vi "IR_OPO_Capture_V2.vi"(0 "Commands array":string[][](array[string])=[["Group20.825", "Group20.671", "Group20.814", "Group30.121"], ["Group2-0.528", "Group2-1.243", "Group2-0.539", "Group30.121"], ["Group20.374", "Group21.573", "Group20.363", "Group30.121"], ["Group2-0.242", "Group2-1.815", "Group2-0.253", "Group30.121"], ["Group20.165", "Group21.991", "Group20.154", "Group30.121"], ["Group2-0.077", "Group2-2.145", "Group2-0.088", "Group30.121"], ["Group20.044", "Group22.233", "Group20.033", "Group30.121"], ["Group2-2.310", "WT10", "WT10", "Group30.121"], ["Group22.310", "WT10", "WT10", "Group30.121"], ["Group2-2.310", "WT10", "WT10", "Group30.121"], ["Group22.310", "WT10", "WT10", "Group30.121"], ["Group2-2.310", "WT10", "WT10", "Group30.121"], ["Group22.310", "WT10", "WT10", "Group30.121"], ["Group2-0.011", "Group2-2.277", "Group2-0.022", "Group30.121"], ["Group20.066", "Group22.189", "Group20.055", "Group30.121"], ["Group2-0.121", "Group2-2.057", "Group2-0.132", "Group30.121"], ["Group20.209", "Group21.903", "Group20.198", "Group30.121"], ["Group2-0.297", "Group2-1.705", "Group2-0.308", "Group30.121"], ["Group20.451", "Group21.419", "Group20.440", "Group30.121"], ["Group2-0.660", "Group2-0.979", "Group2-0.671", "Group30.121"]], 1 "XPS_Address":string="192.168.254.254", 2 "VISA resource name":refnum<visa-resource-name>, 3 "laser array index":i32, 4 "Process time":dbl format="%#_13g", 5 "Axis Speed":dbl=1.0 format="%#_13g", 6 "Laser on/off array":bool[][](array[boolean])=[[FALSE, TRUE, FALSE, FALSE], [FALSE, TRUE, FALSE, FALSE], [FALSE, TRUE, FALSE, FALSE], [FALSE, TRUE, FALSE, FALSE], [FALSE, TRUE, FALSE, FALSE], [FALSE, TRUE, FALSE, FALSE], [FALSE, TRUE, FALSE, FALSE], [TRUE, FALSE, FALSE, FALSE], [TRUE, FALSE, FALSE, FALSE], [TRUE, FALSE, FALSE, FALSE], [TRUE, FALSE, FALSE, FALSE], [TRUE, FALSE, FALSE, FALSE], [TRUE, FALSE, FALSE, FALSE], [FALSE, TRUE, FALSE, FALSE], [FALSE, TRUE, FALSE, FALSE], [FALSE, TRUE, FALSE, FALSE], [FALSE, TRUE, FALSE, FALSE], [FALSE, TRUE, FALSE, FALSE], [FALSE, TRUE, FALSE, FALSE], [FALSE, TRUE, FALSE, FALSE]], 7 "stop":bool, 8 "delay before read (ms)":u32=500, 11 "Axis Initial Parameters":T1={"Velocity (units/seconds)"=1.0, "Acceleration (units/seconds²)"=20.0, "Minimum Jerk Time (seconds)"=0.005, "Maximum Jerk Time (seconds)"=0.009} {"Maximum Jerk Time (seconds)" format="%.6e"; "Minimum Jerk Time (seconds)" format="%.6e"; "Acceleration (units/seconds²)" format="%.6e"; "Velocity (units/seconds)" format="%.6e"}, 13 "ROI Area \n(mm2)":dbl=4.035870075999999, 14 "Axis 2":string="Group3", 15 "Axis 1":string="Group2", 17 "OPO on?":bool, 19 "Acceleration (units/seconds²)":dbl=20.0) -> (10 "Elapsed time":dbl)   [LabVIEW 2016]
uses:
  case selector.ctl
panel:
  out "Capture Log":string
  out "Axis 1 position":dbl format="%.10f"
  out "Axis 2 position":dbl format="%.10f"
  out "Initial time":timestamp
  in  "Active Positioner":string
  out "Current Line":i32
  out "1D Laser Array":bool[](array[boolean])=[FALSE, TRUE, FALSE, FALSE, FALSE, TRUE, FALSE, FALSE, FALSE, TRUE, FALSE, FALSE, FALSE, TRUE, FALSE, FALSE, FALSE, TRUE, FALSE, FALSE, FALSE, TRUE, FALSE, FALSE, FALSE, TRUE, FALSE, FALSE, TRUE, FALSE, FALSE, FALSE, TRUE, FALSE, FALSE, FALSE, TRUE, FALSE, FALSE, FALSE, TRUE, FALSE, FALSE, FALSE, TRUE, FALSE, FALSE, FALSE, TRUE, FALSE, FALSE, FALSE, FALSE, TRUE, FALSE, FALSE, FALSE, TRUE, FALSE, FALSE, FALSE, TRUE, FALSE, FALSE, FALSE, TRUE, FALSE, FALSE, FALSE, TRUE, FALSE, FALSE, FALSE, TRUE, FALSE, FALSE, FALSE, TRUE, FALSE, FALSE]
  out "1D command array":string[](array[string])=["Group20.825", "Group20.671", "Group20.814", "Group30.121", "Group2-0.528", "Group2-1.243", "Group2-0.539", "Group30.121", "Group20.374", "Group21.573", "Group20.363", "Group30.121", "Group2-0.242", "Group2-1.815", "Group2-0.253", "Group30.121", "Group20.165", "Group21.991", "Group20.154", "Group30.121", "Group2-0.077", "Group2-2.145", "Group2-0.088", "Group30.121", "Group20.044", "Group22.233", "Group20.033", "Group30.121", "Group2-2.310", "WT10", "WT10", "Group30.121", "Group22.310", "WT10", "WT10", "Group30.121", "Group2-2.310", "WT10", "WT10", "Group30.121", "Group22.310", "WT10", "WT10", "Group30.121", "Group2-2.310", "WT10", "WT10", "Group30.121", "Group22.310", "WT10", "WT10", "Group30.121", "Group2-0.011", "Group2-2.277", "Group2-0.022", "Group30.121", "Group20.066", "Group22.189", "Group20.055", "Group30.121", "Group2-0.121", "Group2-2.057", "Group2-0.132", "Group30.121", "Group20.209", "Group21.903", "Group20.198", "Group30.121", "Group2-0.297", "Group2-1.705", "Group2-0.308", "Group30.121", "Group20.451", "Group21.419", "Group20.440", "Group30.121", "Group2-0.660", "Group2-0.979", "Group2-0.671", "Group30.121"]
  out "Current Command":string
  out "Current laser element":bool
  out "Total lines":i32=80
  in  "Active Axis":string
  out "Laser on/off":bool
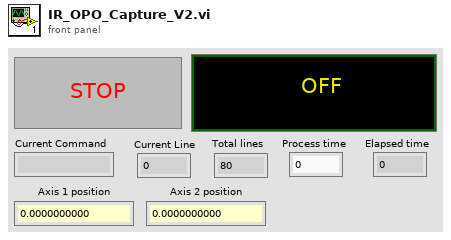
[diagram p1: front panel]
types:
  T1 = cluster{"Velocity (units/seconds)":dbl, "Acceleration (units/seconds²)":dbl, "Minimum Jerk Time (seconds)":dbl, "Maximum Jerk Time (seconds)":dbl}
  T2 = typedef "case selector.ctl" = enum16{"Initialize", "Element selection", "Laser", "Velocities", "Command", "Wait", "Exit"}
  T3 = enum16{"open", "replace", "create", "open or create", "replace or create", "replace or create with confirmation"}
  T4 = cluster{"connection TCP":refnum<k5>, "LogTo File":bool, "Log File refnum":refnum<file>, "no error if error log":bool}
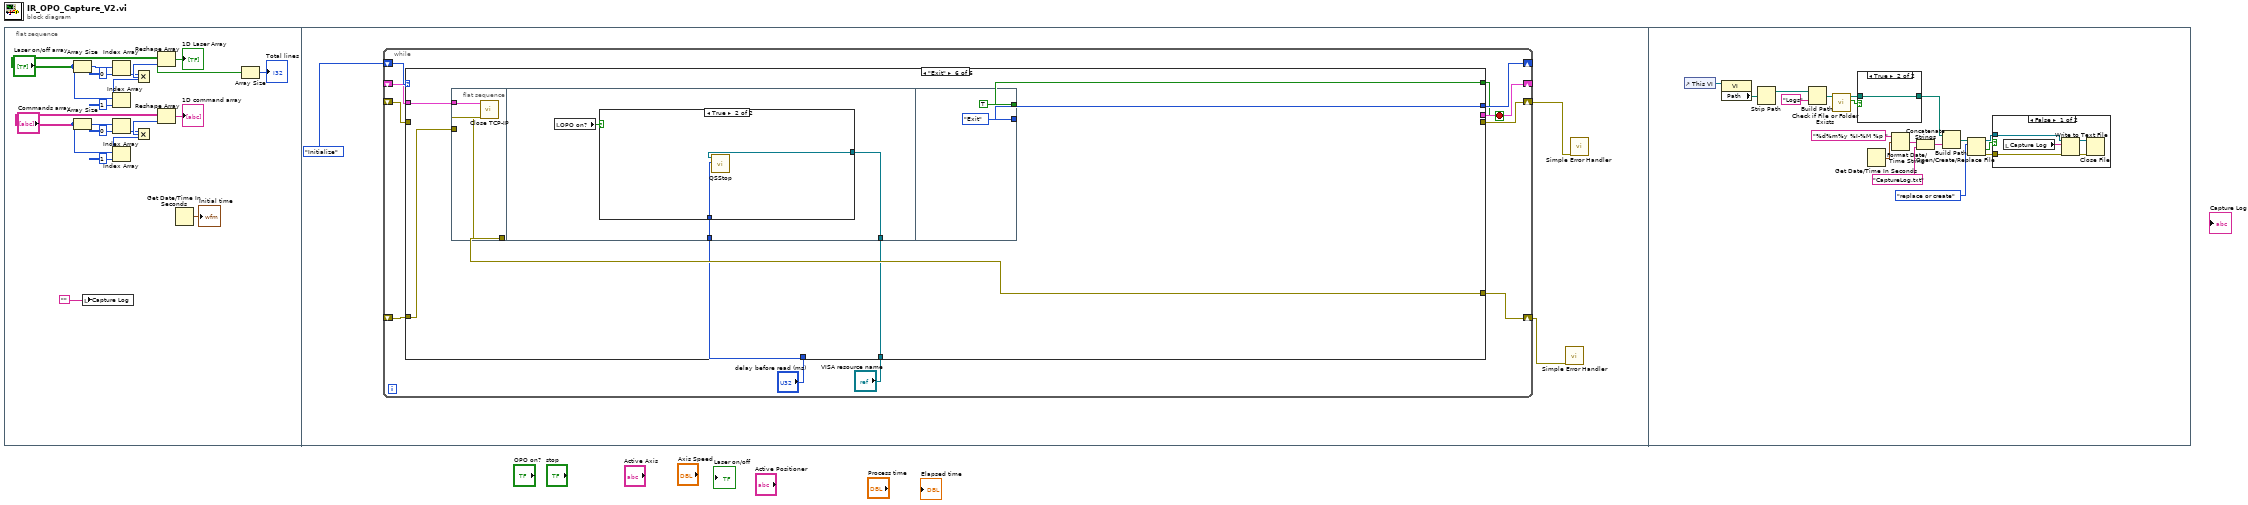
[diagram p0: block diagram]
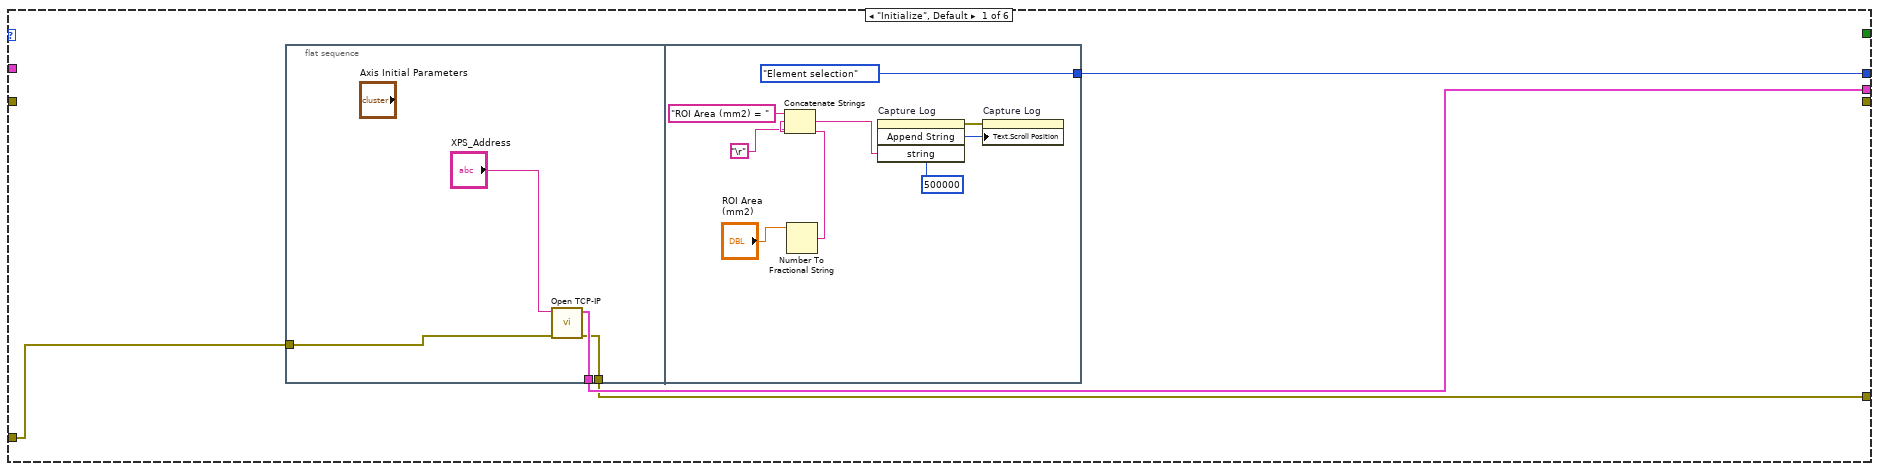
[diagram p2: hidden frame]
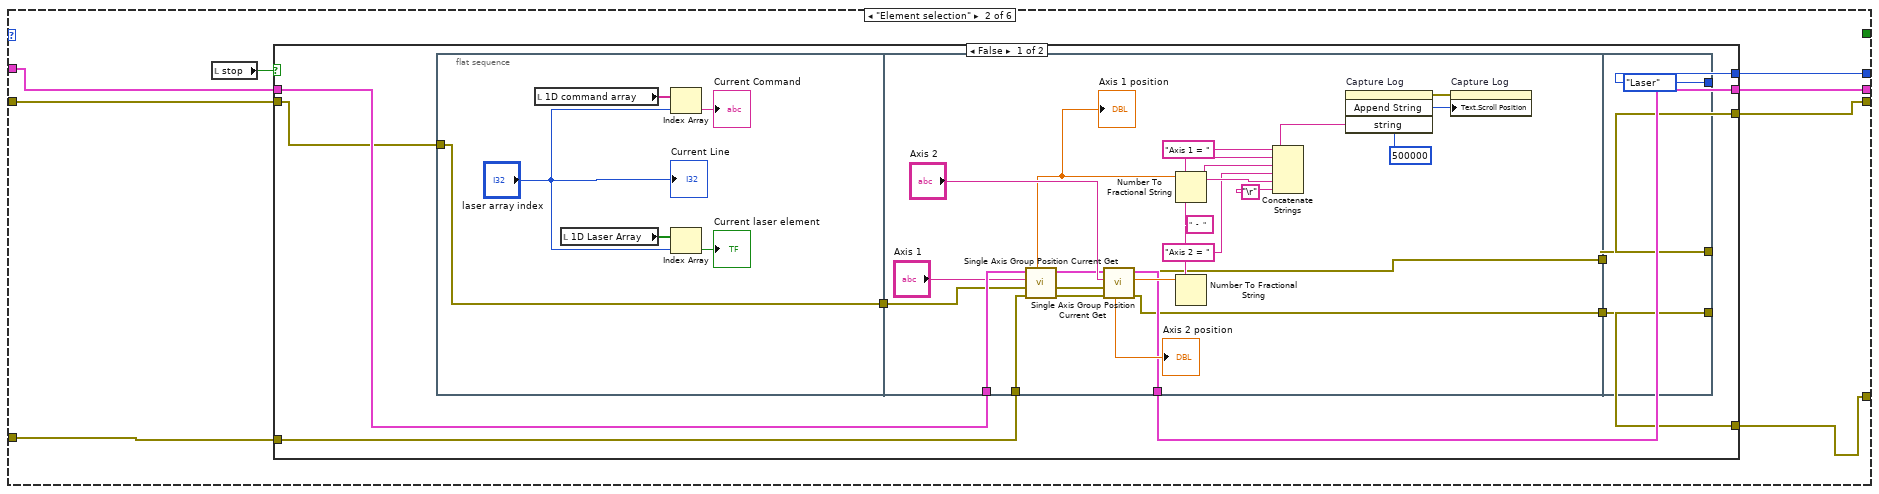
[diagram p3: hidden frame]
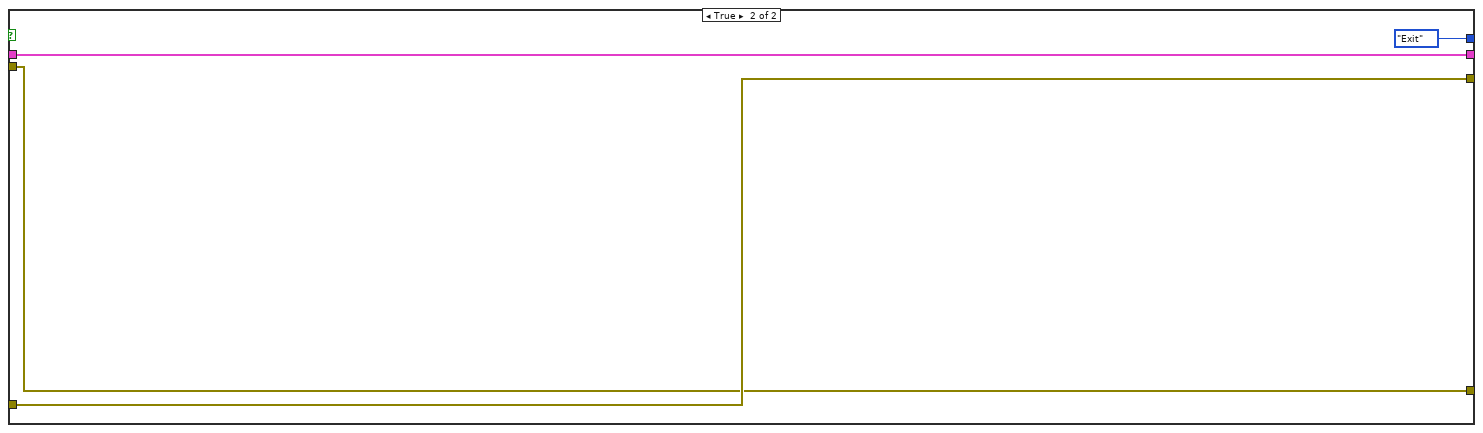
[diagram p4: hidden frame]
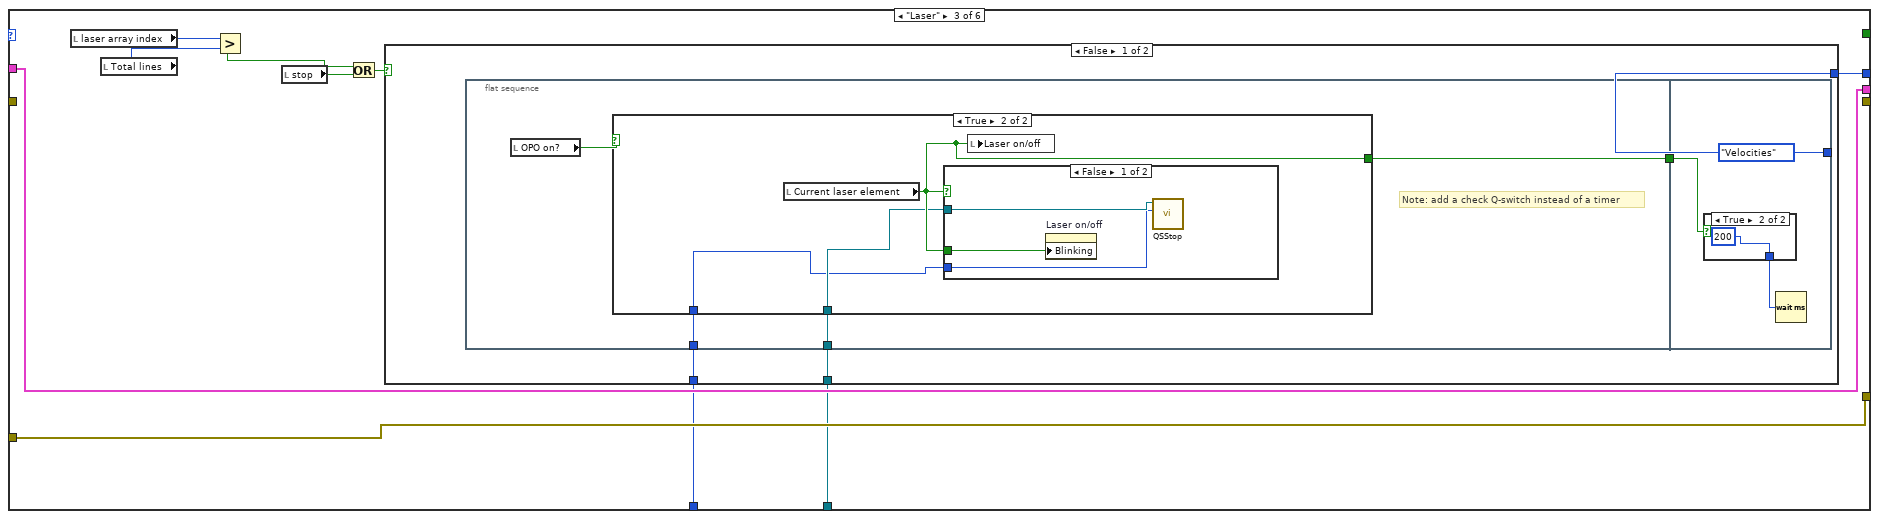
[diagram p5: hidden frame]
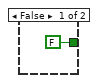
[diagram p6: hidden frame]
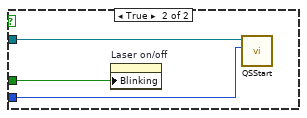
[diagram p7: hidden frame]
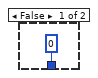
[diagram p8: hidden frame]
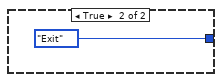
[diagram p9: hidden frame]
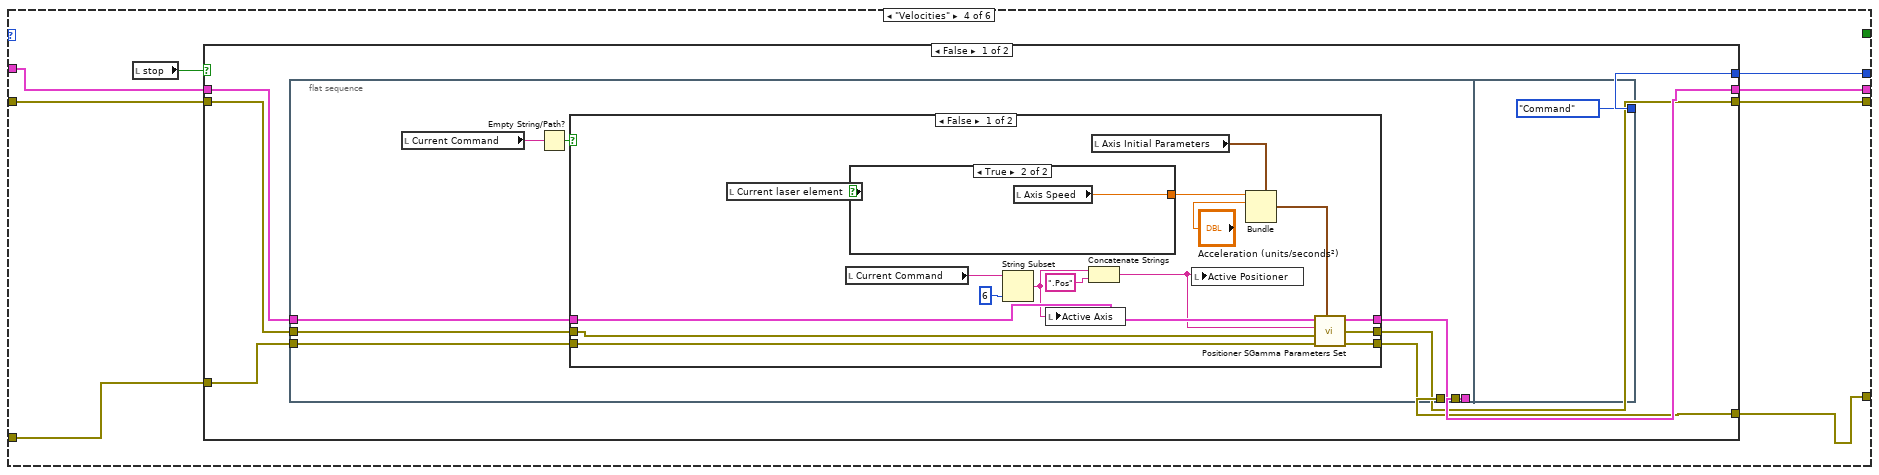
[diagram p10: hidden frame]
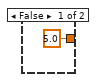
[diagram p11: hidden frame]
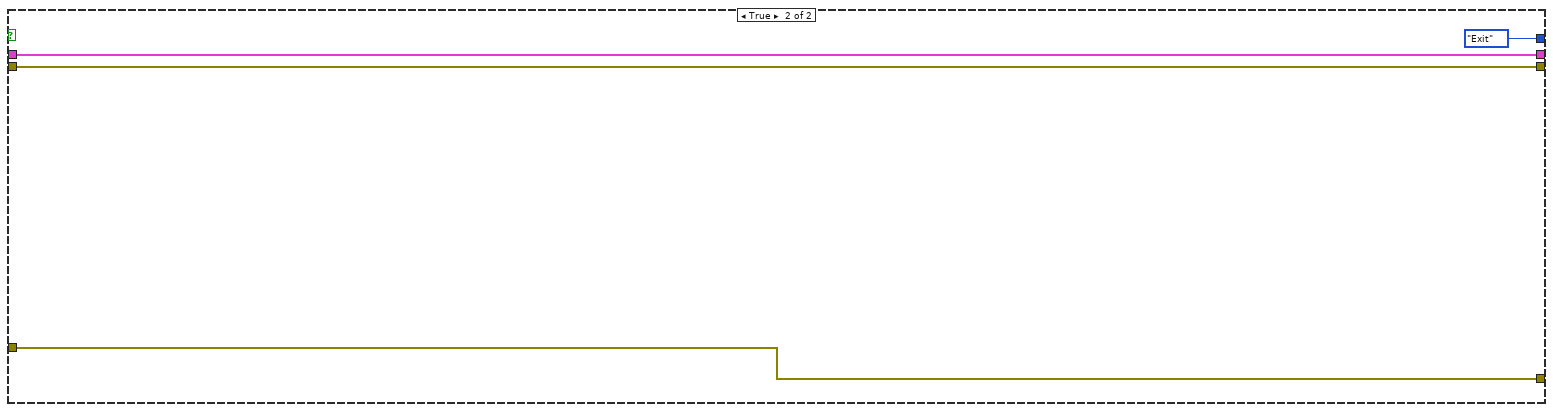
[diagram p13: hidden frame]
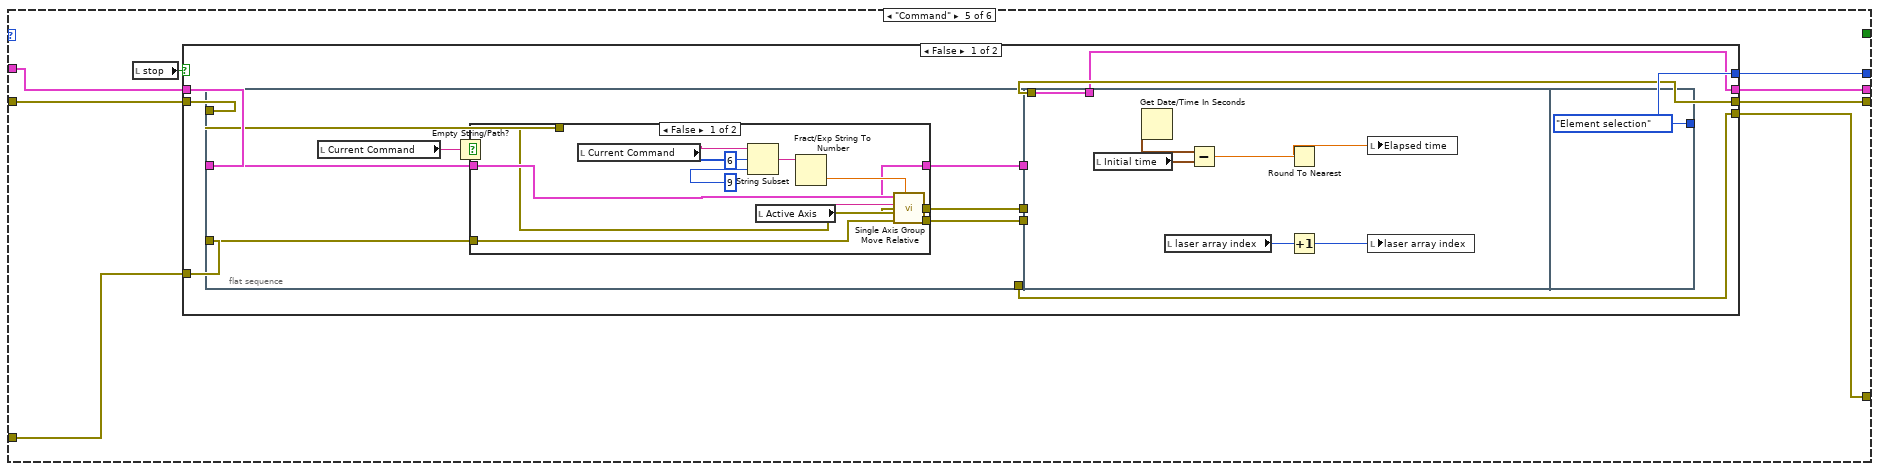
[diagram p14: hidden frame]
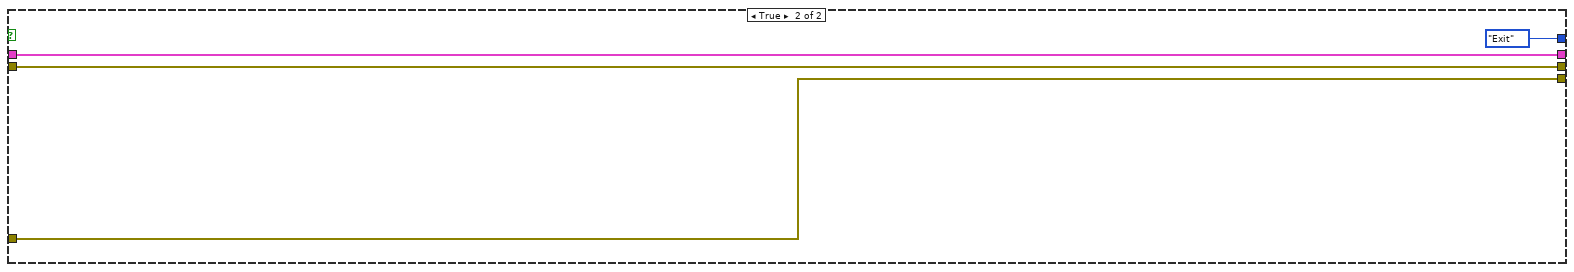
[diagram p16: hidden frame]
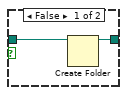
[diagram p18: hidden frame]
diagram:
  n1 = flat-sequence {
    frame #0 {
      n2 = Array Size(array="Laser on/off array") -> (size(s)=w11:i32[])
      n3 = Array Size(array="Commands array") -> (size(s)=w3:i32[])
      n4 = local write "Capture Log"("") -> ()
      n5 = Index Array(array=w11, index=0) -> (element=w14:i32)
      n6 = Index Array(array=w11, index=1) -> (element=w15:i32)
      n7 = Index Array(array=w3, index=0) -> (element=w6:i32)
      n8 = Index Array(array=w3, index=1) -> (element=w7:i32)
      n9 = Multiply(x=w14, y=w15) -> (x*y=w16:i32)
      n10 = Multiply(x=w6, y=w7) -> (x*y=w8:i32)
      n11 = Reshape Array("Laser on/off array", w16) -> (w19:bool[])
      "1D Laser Array" <- w19
      n12 = Reshape Array("Commands array", w8) -> (→"1D command array":string[])
      n13 = Get Date/Time In Seconds() -> (seconds since 1Jan1904=→"Initial time":timestamp)
      n14 = Array Size(array=w19) -> (size(s)=→"Total lines":i32)
    }
    frame #1 {
      n15 = while {
        shift-right: [w32] -> _
        shift-left: case_selector."Initialize" -> [w33]
        shift-right: [w30] -> w20
        shift-left: _ -> [w31]
        shift-right: [w29] -> _
        shift-left: _ -> [w28]
        shift-right: [w27] -> w21
        shift-left: _ -> [w26]
        stop <- w25 stop-if-true
        n16 = case shown="\"Exit\"" w33 {
          tunnel: [w37 w57 w112 w144 w193 w244] -> w32
          tunnel: w31 -> [w36 w54 w111 w142 w191 w245]
          tunnel: [w34 w51 w111 w141 w190 w243] -> w30
          tunnel: [w35 w50 w105 w139 w188 _] -> w29
          tunnel: w28 -> [_ w55 w105 w140 w189 w242]
          tunnel: [_ w52 _ w138 w186 _] -> w27
          tunnel: w26 -> [_ w53 _ w137 w187 _]
          tunnel: [_ _ _ _ _ w241] -> w25
          tunnel: "VISA resource name" -> [_ _ w104 _ _ w239]
          tunnel: "delay before read (ms)" -> [_ _ w103 _ _ w240]
          frame "Initialize", Default {
            n17 = flat-sequence {
              tunnel: w36 -> [w40]
              tunnel: [w39] -> w35
              tunnel: [w38] -> w34
              tunnel: [case_selector."Element selection"] -> w37
              frame #0 {
                n18 = call <userlib>:"Open TCP-IP.vi"("error in (no error)"=w40, "IP address"="XPS_Address") -> ("error out"=w38:errorcluster, "Connection ID"=w39:T4)  [unwired: 7 in, 1 out]
              }
              frame #1 {
                n19 = Number To Fractional String(number="ROI Area \n(mm2)") -> (F-format string=w45:string)  [unwired: 3 in]
                n20 = Concatenate Strings("ROI Area (mm2) = " ("string"), w45, "\r") -> (w43:string)
                n21 = invoke on="Capture Log" class="Str" method="Append String"("string"=w43) -> (error out=w47:errorcluster)  [unwired: 3 in, 3 out]
                n22 = property on="Capture Log" class="Str"(error in=w47, "Text.Scroll Position"=u32 500000) -> ()  [unwired: 1 in, 2 out]
              }
            }
          }
          frame "Element selection" {
            n23 = local read "stop"() -> (w56:bool)
            n24 = case shown="False" w56 {
              tunnel: [w66 case_selector."Exit"] -> w57
              tunnel: w55 -> [w67 w101]
              tunnel: w54 -> [w60 w100]
              tunnel: w53 -> [w59 w99]
              tunnel: [w61 w100] -> w52
              tunnel: [w63 w99] -> w51
              tunnel: [w65 w101] -> w50
              frame False {
                n25 = flat-sequence {
                  tunnel: w59 -> [w68]
                  tunnel: [w68] -> w58
                  tunnel: w67 -> [w86]
                  tunnel: w60 -> [w84]
                  tunnel: [w77] -> w65
                  tunnel: [w76] -> w64
                  tunnel: [w75] -> w62
                  tunnel: w58 -> [w74]
                  tunnel: [case_selector."Laser"] -> w66
                  tunnel: w64 -> [w97]
                  tunnel: [w97] -> w63
                  tunnel: w62 -> [w96]
                  tunnel: [w96] -> w61
                  frame #0 {
                    n26 = local read "1D command array"() -> (w71:string[])
                    n27 = local read "1D Laser Array"() -> (w70:bool[])
                    n28 = Index Array(array=w71, index="laser array index") -> (element=→"Current Command":string)
                    n29 = Index Array(array=w70, index="laser array index") -> (element=→"Current laser element":bool)
                    "Current Line" <- "laser array index"
                  }
                  frame #1 {
                    n30 = call <userlib>:"Single Axis Group Position Current Get.vi"("error in (no error)"=w84, "XPS error in (no error)"=w74, "SingleAxis Group  Name (250 c max)"="Axis 1", "connection ID in"=w86) -> ("error out"=w78:errorcluster, "XPS error out"=w79:errorcluster, "Current Position (units)"=w83:dbl, "connection ID out"=w80:T4)  [unwired: 4 in]
                    "Axis 1 position" <- w83
                    n31 = call <userlib>:"Single Axis Group Position Current Get.vi"("error in (no error)"=w78, "XPS error in (no error)"=w79, "SingleAxis Group  Name (250 c max)"="Axis 2", "connection ID in"=w80) -> ("error out"=w76:errorcluster, "XPS error out"=w75:errorcluster, "Current Position (units)"=w82:dbl, "connection ID out"=w77:T4)  [unwired: 4 in]
                    "Axis 2 position" <- w82
                    n32 = Number To Fractional String(number=w83) -> (F-format string=w94:string)  [unwired: 3 in]
                    n33 = Number To Fractional String(number=w82) -> (F-format string=w92:string)  [unwired: 3 in]
                    n34 = Concatenate Strings("Axis 1 = " ("string"), w94, "  -  " ("string"), "Axis 2 = " ("string"), w92, "\r") -> (w89:string)
                    n35 = invoke on="Capture Log" class="Str" method="Append String"("string"=w89) -> (error out=w88:errorcluster)  [unwired: 3 in, 3 out]
                    n36 = property on="Capture Log" class="Str"(error in=w88, "Text.Scroll Position"=u32 500000) -> ()  [unwired: 1 in, 2 out]
                  }
                  frame #2 {
                  }
                }
              }
              frame True {
              }
            }
          }
          frame "Laser" {
            n37 = local read "laser array index"() -> (w109:i32)
            n38 = local read "Total lines"() -> (w110:i32)
            n39 = Greater?(x=w109, y=w110) -> (0:w107:bool)
            n40 = local read "stop"() -> (w108:bool)
            n41 = Or(x=w107, y=w108) -> (x .or. y?=w106:bool)
            n42 = case shown="False" w106 {
              tunnel: [w116 case_selector."Exit"] -> w112
              tunnel: w104 -> [w114 _]
              tunnel: w103 -> [w113 _]
              frame False {
                n43 = flat-sequence {
                  tunnel: [w119] -> w115
                  tunnel: w114 -> [w118]
                  tunnel: w113 -> [w117]
                  tunnel: [case_selector."Velocities"] -> w116
                  tunnel: w115 -> [w132]
                  frame #0 {
                    # "Note: add a check Q-switch instead of a timer"
                    n44 = local read "OPO on?"() -> (w120:bool)
                    n45 = case shown="True" w120 {
                      tunnel: [FALSE ("Current laser element") w124] -> w119
                      tunnel: w118 -> [_ w123]
                      tunnel: w117 -> [_ w122]
                      frame False {
                      }
                      frame True {
                        n46 = local read "Current laser element"() -> (w124:bool)
                        n47 = case shown="False" w124 {
                          tunnel: w124 -> [w127 w130]
                          tunnel: w123 -> [w126 w129]
                          tunnel: w122 -> [w125 w128]
                          frame False {
                            n48 = property on="Laser on/off" class="Bool (strict)"("Blinking"=w127) -> ()  [unwired: 2 in, 2 out]
                            n49 = call "QSStop.vi"("delay before read (ms)"=w125, "VISA resource name"=w126) -> ()  [unwired: 6 in, 4 out]
                          }
                          frame True {
                            n50 = property on="Laser on/off" class="Bool (strict)"("Blinking"=w130) -> ()  [unwired: 2 in, 2 out]
                            n51 = call "QSStart.vi"("delay before read (ms)"=w128, "VISA resource name"=w129) -> ()  [unwired: 6 in, 4 out]
                          }
                        }
                        n52 = local write "Laser on/off"(w124) -> ()
                      }
                    }
                  }
                  frame #1 {
                    n53 = case shown="True" w132 {
                      tunnel: [u32 0 ("milliseconds to wait") u32 200 ("milliseconds to wait")] -> w131
                      frame False {
                      }
                      frame True {
                      }
                    }
                    n54 = Wait (ms)(milliseconds to wait=w131) -> ()  [unwired: 1 out]
                  }
                }
              }
              frame True {
              }
            }
          }
          frame "Velocities" {
            n55 = local read "stop"() -> (w143:bool)
            n56 = case shown="False" w143 {
              tunnel: [w151 case_selector."Exit"] -> w144
              tunnel: w142 -> [w150 w184]
              tunnel: [w147 w184] -> w141
              tunnel: w140 -> [w149 w183]
              tunnel: [w148 w183] -> w139
              tunnel: [w146 w182] -> w138
              tunnel: w137 -> [w145 w182]
              frame False {
                n57 = flat-sequence {
                  tunnel: w150 -> [w157]
                  tunnel: w149 -> [w159]
                  tunnel: [w158] -> w148
                  tunnel: [w156] -> w147
                  tunnel: [w155] -> w146
                  tunnel: w145 -> [w154]
                  tunnel: [case_selector."Command"] -> w151
                  frame #0 {
                    n58 = local read "Current Command"() -> (w153:string)
                    n59 = Empty String/Path?(string/path=w153) -> (empty?=w152:bool)
                    n60 = case shown="False" w152 {
                      tunnel: w159 -> [w172 w178]
                      tunnel: [w171 w178] -> w158
                      tunnel: w157 -> [w170 w179]
                      tunnel: [w169 w179] -> w156
                      tunnel: [w164 w180] -> w155
                      tunnel: w154 -> [w163 w180]
                      frame False {
                        n61 = local read "Current laser element"() -> (w175:bool)
                        n62 = local read "Current Command"() -> (w173:string)
                        n63 = case shown="True" w175 {
                          tunnel: [5.0 w177] -> w168
                          frame False {
                          }
                          frame True {
                            n64 = local read "Axis Speed"() -> (w177:dbl)
                          }
                        }
                        n65 = String Subset(string=w173, length (rest)=6 ("length (rest)")) -> (substring=w162:string)  [unwired: 1 in]
                        n66 = local write "Active Axis"(w162) -> ()
                        n67 = Concatenate Strings(w162, ".Pos" ("string")) -> (w161:string)
                        n68 = local read "Axis Initial Parameters"() -> (w166:T1)
                        n69 = local write "Active Positioner"(w161) -> ()
                        n70 = Bundle(cluster=w166, "Velocity (units/seconds)"=w168, "Acceleration (units/seconds²)"="Acceleration (units/seconds²)") -> (w167:T1)  [unwired: 2 in]
                        n71 = call <userlib>:"Positioner SGamma Parameters Set.vi"("SGamma Parameters"=w167, "error in (no error)"=w170, "XPS error in (no error)"=w163, "Positioner Name (250 c max)"=w161, "connection ID in"=w172) -> ("error out"=w169:errorcluster, "XPS error out"=w164:errorcluster, "connection ID out"=w171:T4)  [unwired: 4 in]
                      }
                      frame True {
                      }
                    }
                  }
                  frame #1 {
                  }
                }
              }
              frame True {
              }
            }
          }
          frame "Command" {
            n72 = local read "stop"() -> (w192:bool)
            n73 = case shown="False" w192 {
              tunnel: [w197 case_selector."Exit"] -> w193
              tunnel: w191 -> [w201 w237]
              tunnel: [w195 w237] -> w190
              tunnel: w189 -> [w203 w236]
              tunnel: [w194 w236] -> w188
              tunnel: w187 -> [w200 w235]
              tunnel: [w196 w235] -> w186
              frame False {
                n74 = flat-sequence {
                  tunnel: w203 -> [w211]
                  tunnel: [w210] -> w202
                  tunnel: w201 -> [w207]
                  tunnel: w200 -> [w206]
                  tunnel: [w205] -> w199
                  tunnel: [w204] -> w198
                  tunnel: w202 -> [w225]
                  tunnel: w199 -> [w227]
                  tunnel: w198 -> [w226]
                  tunnel: [w227] -> w196
                  tunnel: [w226] -> w195
                  tunnel: [w225] -> w194
                  tunnel: [case_selector."Element selection"] -> w197
                  frame #0 {
                    n75 = local read "Current Command"() -> (w208:string)
                    n76 = Empty String/Path?(string/path=w208) -> (empty?=w209:bool)
                    n77 = case shown="False" w209 {
                      tunnel: w211 -> [w223 w224]
                      tunnel: [w216 w224] -> w210
                      tunnel: w207 -> [w215 _]
                      tunnel: w206 -> [w214 _]
                      tunnel: [w213 _] -> w205
                      tunnel: [w212 _] -> w204
                      frame False {
                        n78 = local read "Current Command"() -> (w222:string)
                        n79 = String Subset(string=w222, offset (0)=6, length (rest)=9 ("length (rest)")) -> (substring=w219:string)
                        n80 = local read "Active Axis"() -> (w217:string)
                        n81 = Fract/Exp String To Number(string=w219) -> (number=w218:dbl)  [unwired: 3 in, 1 out]
                        n82 = call <userlib>:"Single Axis Group Move Relative.vi"("Target Displacement (units)"=w218, "error in (no error)"=w215, "XPS error in (no error)"=w214, "SingleAxis Group  Name (250 c max)"=w217, "connection ID in"=w223) -> ("error out"=w212:errorcluster, "XPS error out"=w213:errorcluster, "connection ID out"=w216:T4)  [unwired: 4 in]
                      }
                      frame True {
                      }
                    }
                  }
                  frame #1 {
                    n83 = local read "Initial time"() -> (w230:timestamp)
                    n84 = Get Date/Time In Seconds() -> (seconds since 1Jan1904=w231:timestamp)
                    n85 = local read "laser array index"() -> (w233:i32)
                    n86 = Subtract(x=w231, y=w230) -> (x-y=w229:dbl)
                    n87 = Round To Nearest(number=w229) -> (nearest integer value=w228:dbl)
                    n88 = Increment(x=w233) -> (x+1=w232:i32)
                    n89 = local write "Elapsed time"(w228) -> ()
                    n90 = local write "laser array index"(w232) -> ()
                  }
                  frame #2 {
                  }
                }
              }
              frame True {
              }
            }
          }
          frame "Exit" {
            n91 = flat-sequence {
              tunnel: w245 -> [w247]
              tunnel: [w246] -> w243
              tunnel: w242 -> [w248]
              tunnel: w240 -> [w250]
              tunnel: w239 -> [w249]
              tunnel: [case_selector."Exit"] -> w244
              tunnel: [TRUE] -> w241
              frame #0 {
                n92 = call <userlib>:"Close TCP-IP.vi"("error in (no error)"=w247, "connection ID in"=w248) -> ("Error out"=w246:errorcluster)  [unwired: 9 in]
              }
              frame #1 {
                n93 = local read "OPO on?"() -> (w251:bool)
                n94 = case shown="True" w251 {
                  tunnel: w250 -> [_ w253]
                  tunnel: w249 -> [_ w252]
                  frame False {
                  }
                  frame True {
                    n95 = call "QSStop.vi"("delay before read (ms)"=w253, "VISA resource name"=w252) -> ()  [unwired: 6 in, 4 out]
                  }
                }
              }
              frame #2 {
              }
            }
          }
        }
      }
      n96 = call <vilib>:"Simple Error Handler.vi"("error in (no error)"=w20) -> ()  [unwired: 4 in, 5 out]
      n97 = call <vilib>:"Simple Error Handler.vi"("error in (no error)"=w21) -> ()  [unwired: 4 in, 5 out]
    }
    frame #2 {
      n98 = control-ref of="This VI"() -> (w273:refnum<vi>)
      n99 = property class="VI"(reference=w273) -> ("Path"=w272:path)  [unwired: 1 in, 2 out]
      n100 = Strip Path(path=w272) -> (stripped path=w263:path)  [unwired: 1 out]
      n101 = Build Path(base path=w263, name or relative path="Logs") -> (appended path=w265:path)
      n102 = call <vilib>:"Check if File or Folder Exists.vi"("path"=w265) -> ("file or folder exists?"=w264:bool, "dup path"=w262:path)  [unwired: 8 in, 1 out]
      n103 = case shown="True" w264 {
        tunnel: w262 -> [w275 w276]
        tunnel: [w274 w276] -> w259
        frame False {
          n104 = Create Folder(path (use dialog)=w275) -> (created path=w274:path)  [unwired: 2 in, 2 out]
        }
        frame True {
        }
      }
      n105 = Get Date/Time In Seconds() -> (seconds since 1Jan1904=w268:timestamp)
      n106 = Format Date/Time String(time format string (%c)="%d%m%y %I-%M %p ", seconds (now)=w268) -> (date/time string=w270:string)  [unwired: 1 in]
      n107 = Concatenate Strings(w270, "CaptureLog.txt") -> (w260:string)
      n108 = Build Path(base path=w259, name or relative path=w260) -> (appended path=w261:path)
      n109 = Open/Create/Replace File(file path (use dialog)=w261, operation (0:open)=T3."replace or create") -> (refnum out=w258:refnum<file>, cancelled=w256:bool, error out=w257:errorcluster)  [unwired: 4 in]
      n110 = case shown="False" w256 {
        tunnel: w258 -> [w281 _]
        tunnel: w257 -> [w279 _]
        frame False {
          n111 = local read "Capture Log"() -> (w280:string)
          n112 = Write to Text File(file (use dialog)=w281, text=w280, error in=w279) -> (refnum out=w278:refnum<file>, error out=w277:errorcluster)  [unwired: 2 out]
          n113 = Close File(refnum=w278, error in=w277) -> ()  [unwired: 2 out]
        }
        frame True {
        }
      }
    }
  }
